vi "DB Export Action - Export Parameters.vi"(8 "error in (no error)":errorcluster, 10 "selected path":path, 11 "Item Ref in":T1 format="%.0x") -> (0 "error out":errorcluster, 1 "Parm File Path":path, 2 "selected path out":path caption="selected path", 3 "Item Ref out":T1 format="%.0x")   [LabVIEW 2013, in "AIT 664 Custom Device.lvlib"]
uses:
  AIT 664 Custom Device.lvlib
  <vilib>/NI Veristand/Custom Device API/Custom Device Item Ref.ctl
  <vilib>/NI Veristand/Custom Device API/Custom Device API.lvlib
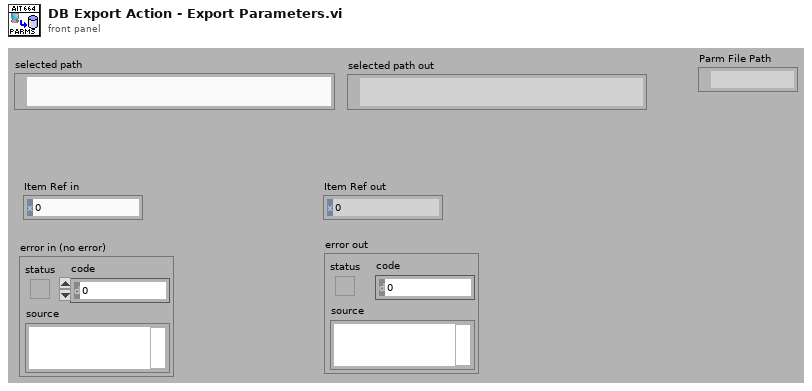
[diagram p1: front panel]
types:
  T1 = typedef "Custom Device API.lvlib/Custom Device Item Ref.ctl" = u64
  T2 = typedef "AIT 664 Custom Device.lvlib/664 - XML Device Description.ctl" = cluster{"Name":string, "Network Speed":string, "MAC Address":string, "VISA Resource Name":string, "End Systems":T3[]}
  T3 = typedef "AIT 664 Custom Device.lvlib/664 - XML End System Description.ctl" = cluster{"Name":string, "Id":u32, "MAC Address":string, "Output VLs":T4[], "Input VLs":T8[]}
  T4 = typedef "AIT 664 Custom Device.lvlib/664 - XML Output VL.ctl" = cluster{"Name":string, "VL Id":u32, "Tx Message Ports":T5[]}
  T5 = typedef "AIT 664 Custom Device.lvlib/664 - XML Tx Message Port.ctl" = cluster{"Name":string, "Port Id":u32, "Sampling Type":T6, "Parameters":T7[], "Source IP Address":string, "Source UDP Port":u32, "Destination IP Address":string, "Destination UDP Port":u32, "Tx Rate (ms)":u32}
  T6 = typedef "AIT 664 Custom Device.lvlib/664 - Sampling Type.ctl" = enum16{"Com Udp", "Com Udp Queuing", "Sap Udp", "Sap Ip", "Sap Mac", "Unknown"}
  T7 = typedef "AIT 664 Custom Device.lvlib/664 -Param.ctl" = cluster{"name":string, "firstByte":i32, "startBit":i32, "numberBits":i32, "scaleFactor":dbl, "scaleOffset":dbl, "signed":bool}
  T8 = typedef "AIT 664 Custom Device.lvlib/664 - XML Input VL.ctl" = cluster{"Name":string, "VL Id":u32, "Rx Message Ports":T9[]}
  T9 = typedef "AIT 664 Custom Device.lvlib/664 - XML Rx Message Port.ctl" = cluster{"Name":string, "Port Id":u32, "Sampling Type":T6, "Parameters":T7[], "Source IP Address":string, "Source UDP Port":u32, "Destination IP Address":string, "Destination UDP Port":u32, "Rx Rate (ms)":u32, "Buffer Depth":u32}
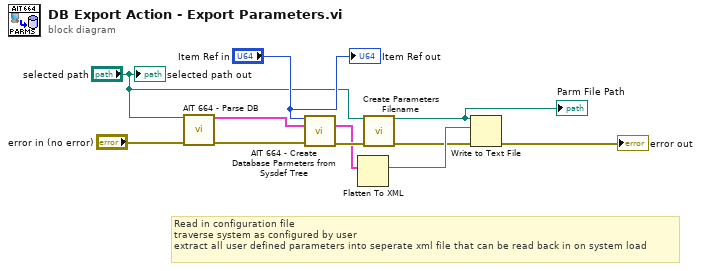
[diagram p0: block diagram]
diagram:
  # "Read in configuration file\ntraverse system as configured by user\nextract all user defined parameters into seperate xml file that can be read back in on system load"
  n1 = call "AIT 664 - Parse DB.vi"("Path in"="selected path", "error in (no error)"="error in (no error)") -> ("664 Device"=w10:T2, "error out"=w9:errorcluster)  [unwired: 12 in]
  n2 = call "AIT 664 - Create Database Parmeters from Sysdef Tree.vi"("Device Ptr"="Item Ref in", "664 Device"=w10, "error in"=w9) -> ("664 Device"=w3:T2, "error out"=w4:errorcluster)  [unwired: 11 in]
  n3 = Flatten To XML(anything=w3) -> (xml string=w2:string)
  n4 = call "Create Parameters Filename.vi"("Simulyzer File Path"="selected path", "error in (no error)"=w4) -> ("Parm File Path"=w5:path, "error out"=w1:errorcluster)  [unwired: 12 in]
  "Parm File Path" <- w5
  n5 = Write to Text File(file (use dialog)=w5, text=w2, error in=w1) -> (error out=→"error out":errorcluster)  [unwired: 1 in, 2 out]
  "Item Ref out" <- "Item Ref in"
  "selected path out" <- "selected path"
